vi "Init Hardware.vi"(8 "error in (no error)":errorcluster, 11 "Andeen-Hagerling Driver in":refnum<class "Andeen-Hagerling Driver.lvclass">) -> (0 "error out":errorcluster, 3 "Andeen-Hagerling Driver out":refnum<class "Andeen-Hagerling Driver.lvclass">)   [LabVIEW 2016, in "Andeen-Hagerling Driver.lvclass"]
uses:
  Andeen-Hagerling Driver.lvclass
  C:/github/NHMFL_Core/Libraries/Instruments/Instrument Driver/Instrument Driver.lvclass
  Instrument Driver/Instrument Driver.lvclass/Instrument Driver.ctl
  Instrument Driver/Read Recorder name.vi
  Instrument Driver/Write Channel names.vi
  Instrument Driver/Write Channel units.vi
  Simple VISA Reader/Simple VISA Reader Driver.lvclass
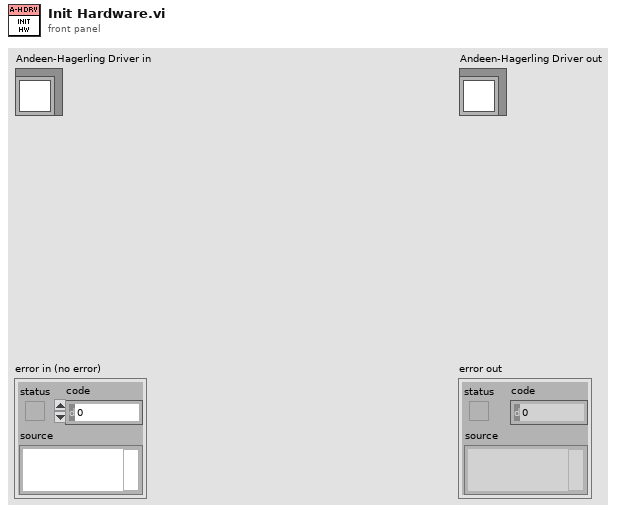
[diagram p1: front panel]
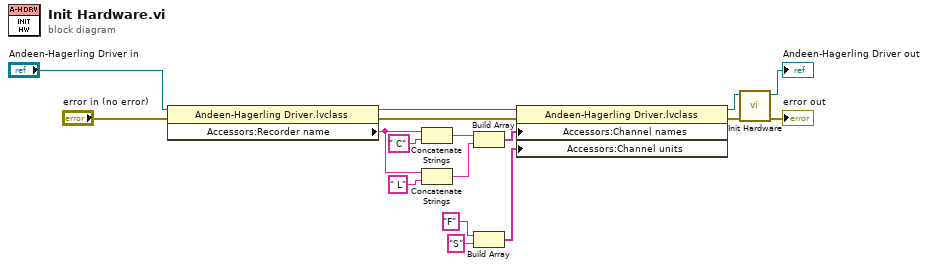
[diagram p0: block diagram]
diagram:
  n1 = property class="Andeen-Hagerling Driver.lvclass"(reference="Andeen-Hagerling Driver in", error in="error in (no error)") -> (reference out=w7:refnum<class "Andeen-Hagerling Driver.lvclass">, error out=w6:errorcluster, "Accessors:Recorder name"=w12:string)
  n2 = Concatenate Strings(w12, " C") -> (w11:string)
  n3 = Concatenate Strings(w12, " L") -> (w14:string)
  n4 = Build Array(w11, w14) -> (w9:string[])
  n5 = Build Array("F", "S" ("element")) -> (w8:string[])
  n6 = property class="Andeen-Hagerling Driver.lvclass"(reference=w7, error in=w6, "Accessors:Channel names"=w9, "Accessors:Channel units"=w8) -> (reference out=w4:refnum<class "Andeen-Hagerling Driver.lvclass">, error out=w2:errorcluster)
  n7 = call-parent "Init Hardware.vi"("error in (no error)"=w2, "Instrument Driver in"=w4) -> ("error out"=→"error out":errorcluster, "Instrument Driver out"=→"Andeen-Hagerling Driver out":refnum<class "Andeen-Hagerling Driver.lvclass">)  [unwired: 8 in]
